vi "Set Channel Threshold.vi"(6 "Threshold state?":bool, 7 "Threshold S1/S2":u16(ring) items=["S1", "S2"], 8 "error in (no error)":errorcluster, 9 "Threshold value (in actual channel unit)":dbl, 10 "Channel":u16(ring) items=["A1"=0, "A2"=1, "A3"=2, "A4"=3, "A5"=4, "A6"=5, "A7"=6, "A8"=7, "A9"=8, "A10"=9, "K1"=200, "K2"=201, "K3"=202, "K4"=203, "FA1"=204, "FA2"=205, "FA3"=206, "FA4"=207], 11 "VISA resource name":refnum<visa-resource-name>) -> (0 "error out":errorcluster, 3 "VISA resource name out":refnum<visa-resource-name>)   [LabVIEW 2017, in "Sefram DAS220.lvlib"]
doc: "Set a channel threashold to display a line on a graphic and setup a trigger level for triggering features.\nThe current channel type defines the unit. (if voltage, consider Volt unit)"
uses:
  <instrlib>/Sefram DAS220/Sefram DAS220.lvlib
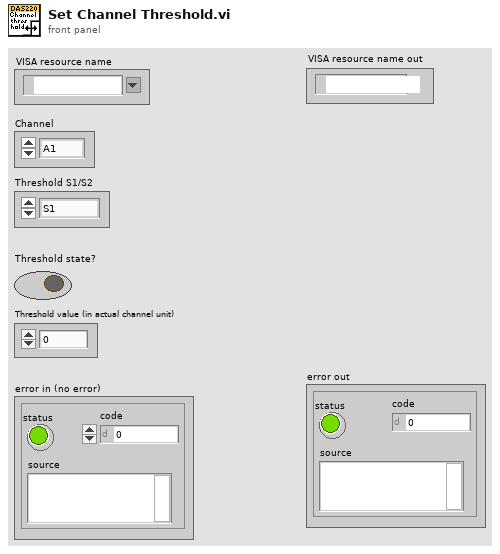
[diagram p1: front panel]
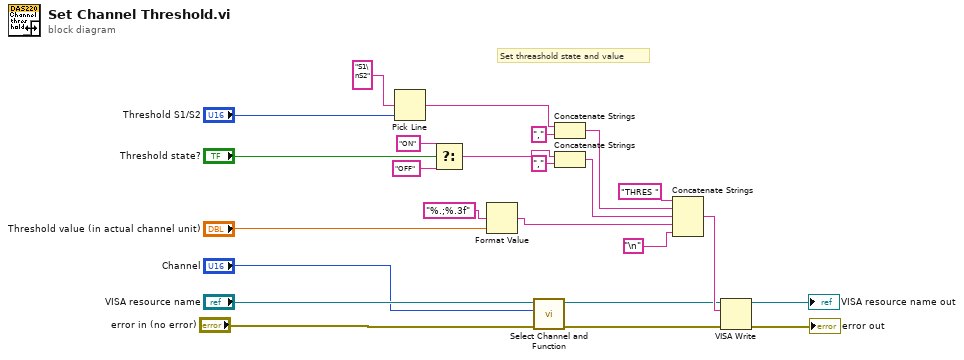
[diagram p0: block diagram]
diagram:
  # "Set threashold state and value"
  n1 = Pick Line(multi-line string="S1\nS2", line index="Threshold S1/S2") -> (output string=w4:string)  [unwired: 1 in]
  n2 = Select(t="ON" ("string"), s="Threshold state?", f="OFF" ("string")) -> (s? t:f=w10:string)
  n3 = Format Value(format string="%.;%.3f", value (0)="Threshold value (in actual channel unit)") -> (output string=w9:string)  [unwired: 1 in]
  n4 = call <instrlib>:"Select Channel and Function.vi"("error in (no error)"="error in (no error)", "Channel"="Channel", "VISA resource name"="VISA resource name") -> ("error out"=w6:errorcluster, "VISA resource name out"=w7:refnum<visa-resource-name>)  [unwired: 7 in]
  n5 = Concatenate Strings(w4, "," ("string")) -> (w20:string)
  n6 = Concatenate Strings(w10, "," ("string")) -> (w18:string)
  n7 = Concatenate Strings("THRES " ("string"), w20, w18, w9, "\n") -> (w24:string)
  n8 = VISA Write(VISA resource name=w7, write buffer=w24, error in (no error)=w6) -> (VISA resource name out=→"VISA resource name out":refnum<visa-resource-name>, error out=→"error out":errorcluster)  [unwired: 1 out]
